vi "RIO Control.vi"() -> (0 "Disable Sensors":bool, 1 "Lift Control":bool, 2 "4Bar Control":bool, 3 "Joystick Value":dbl, 4 "Grabber Inhale":bool, 5 "Grabber Exhale":bool, 6 "Close Gripper":bool, 7 "Open Gripper":bool, 8 "Jaw Open":bool, 9 "Jaw Close":bool)   [LabVIEW 2014]
uses:
  <vilib>/Rock Robotics/WPI/Joystick/WPI_JoystickGetSetRefNum.vi
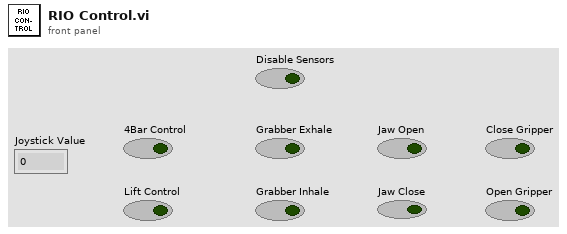
[diagram p1: front panel]
types:
  T1 = typedef "WPI_JoystickDevRef.ctl" = cluster{"Device":T2}
  T2 = typedef "WPI_JoystickDeviceEnum.ctl" = enum16{"USB 0", "USB 1", "USB 2", "USB 3", "USB 4", "USB 5"}
  T3 = cluster{"Axes[0]":dbl, "Axes[1]":dbl, "Axes[2]":dbl, "Axes[3]":dbl, "Axes[4]":dbl, "Axes[5]":dbl, "Axes[6]":dbl, "Axes[7]":dbl, "Axes[8]":dbl}
  T4 = cluster{"Buttons[0]":bool, "Buttons[1]":bool, "Buttons[2]":bool, "Buttons[3]":bool, "Buttons[4]":bool, "Buttons[5]":bool, "Buttons[6]":bool, "Buttons[7]":bool, "Buttons[8]":bool, "Buttons[9]":bool, "Buttons[10]":bool}
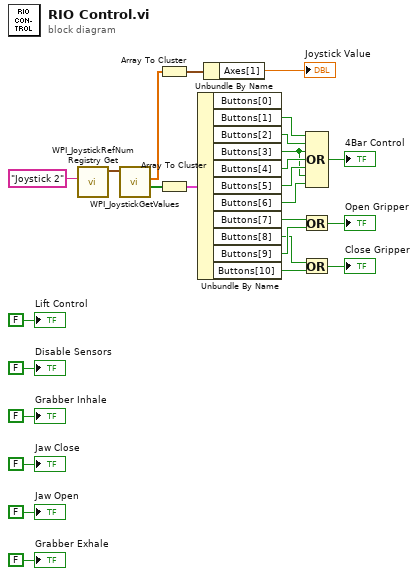
[diagram p0: block diagram]
diagram:
  n1 = call <vilib>:"WPI_JoystickRefNum Registry Get.vi"("refnum name"="Joystick 2") -> ("JoystickDevRef"=w23:T1)  [unwired: 1 in, 9 out]
  n2 = call <vilib>:"WPI_JoystickGetValues.vi"("JoystickDevRef"=w23) -> ("Buttons"=w21:bool[], "Axes"=w24:dbl[])  [unwired: 6 in, 3 out]
  n3 = Array To Cluster(array=w24) -> (cluster=w25:T3)
  n4 = Array To Cluster(array=w21) -> (cluster=w20:T4)
  n5 = Unbundle By Name(w20) -> ("Buttons[1]"=w15:bool, "Buttons[2]"=w14:bool, "Buttons[3]"=w10:bool, "Buttons[4]"=w13:bool, "Buttons[5]"=w12:bool, "Buttons[6]"=w9:bool, "Buttons[7]"=w6:bool, "Buttons[8]"=w3:bool, "Buttons[9]"=w5:bool, "Buttons[10]"=w2:bool)  [unwired: 1 out]
  n6 = Unbundle By Name(w25) -> ("Axes[1]"=→"Joystick Value":dbl)
  n7 = Or(x=w6, y=w5) -> (x .or. y?=→"Open Gripper":bool)
  n8 = Or(x=w3, y=w2) -> (x .or. y?=→"Close Gripper":bool)
  n9 = Compound Arithmetic op=OR(w15, w14, w10, w13, w12, w10, w9) -> (→"4Bar Control":bool)
  "Grabber Exhale" <- FALSE ("Grabber Exhale")
  "Grabber Inhale" <- FALSE ("Grabber Inhale")
  "Lift Control" <- FALSE ("Lift Control")
  "Jaw Open" <- FALSE ("Jaw Open")
  "Jaw Close" <- FALSE ("Jaw Close")
  "Disable Sensors" <- FALSE ("Disable Sensors")
